vi "CRYExport TextFormat.vi"(8 "sAction":string, 11 "Type (data)":enum16{"data", "results"}(ring)) -> (0 "Canceled":bool, 3 "Export format":T1)   [LabVIEW 2013]
uses:
  CRYMainGlobal.vi
panel:
  out "Notation Frame":bool caption="符号"
  out "Layout Frame":bool caption="布局"
  out "Header":bool caption="页眉"
  out "Axes Saved":bool caption="保存的轴"
  in  "save z":bool
  in  "save y":bool
  in  "save x":bool
  in  "Comment":string caption="评论"
  in  "cancel":bool
  in  "save as":bool
  in  "Decimal places":i32=2 caption="小数位"
  in  "Custom Header":string caption="自定义页眉"
  in  "Character":string caption="字符"
  in  "Delimiter":i32(ring) caption="分隔符" items=["tab", "comma", "space", "other"]
  in  "notation":u16(slide) caption="Notation"
  in  "Layout":u16(slide)
  in  "Header format":u16(slide) caption="Header"
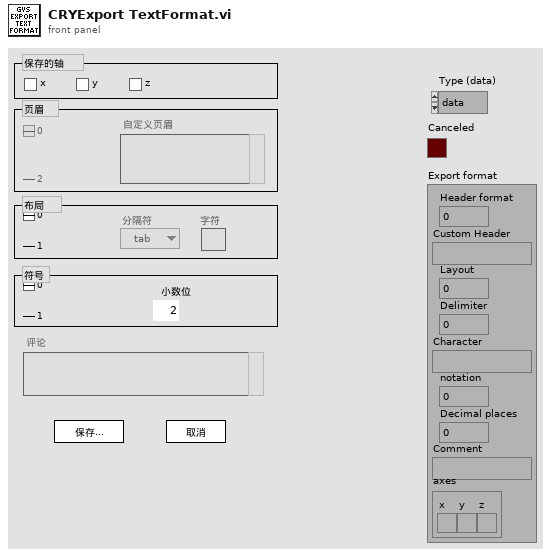
[diagram p1: front panel]
types:
  T1 = cluster{"Header format":u16, "Custom Header":string, "Layout":u16, "Delimiter":i32, "Character":string, "notation":u16, "Decimal places":i32, "Comment":string, "axes":cluster{"x":bool, "y":bool, "z":bool}}
  T2 = enum16{"open", "open or create", "create or replace", "create"}
  T3 = cluster{"Header format":u16, "Custom Header":string, "Layout":u16, "Delimiter":i32, "Character":string, "notation":u16, "Decimal places":i32, "Comment":string}
  T4 = enum8{"Enabled", "Disabled", "Disabled and Grayed Out"}
  T5 = cluster{"Header format":u16, "Custom Header":string, "Layout":u16, "Delimiter":i32, "Character":string, "notation":u16, "Decimal places":i32, "Comment":string, "axes":cluster{"x":bool, "y":bool, "z":bool}}[]
  T6 = cluster{"save x":bool, "save y":bool, "save z":bool}
  T7 = cluster{"Header format":u16, "Custom Header":string, "Layout":u16, "Delimiter":i32, "Character":string, "notation":u16, "Decimal places":i32, "Comment":string, cluster{"save x":bool, "save y":bool, "save z":bool}}
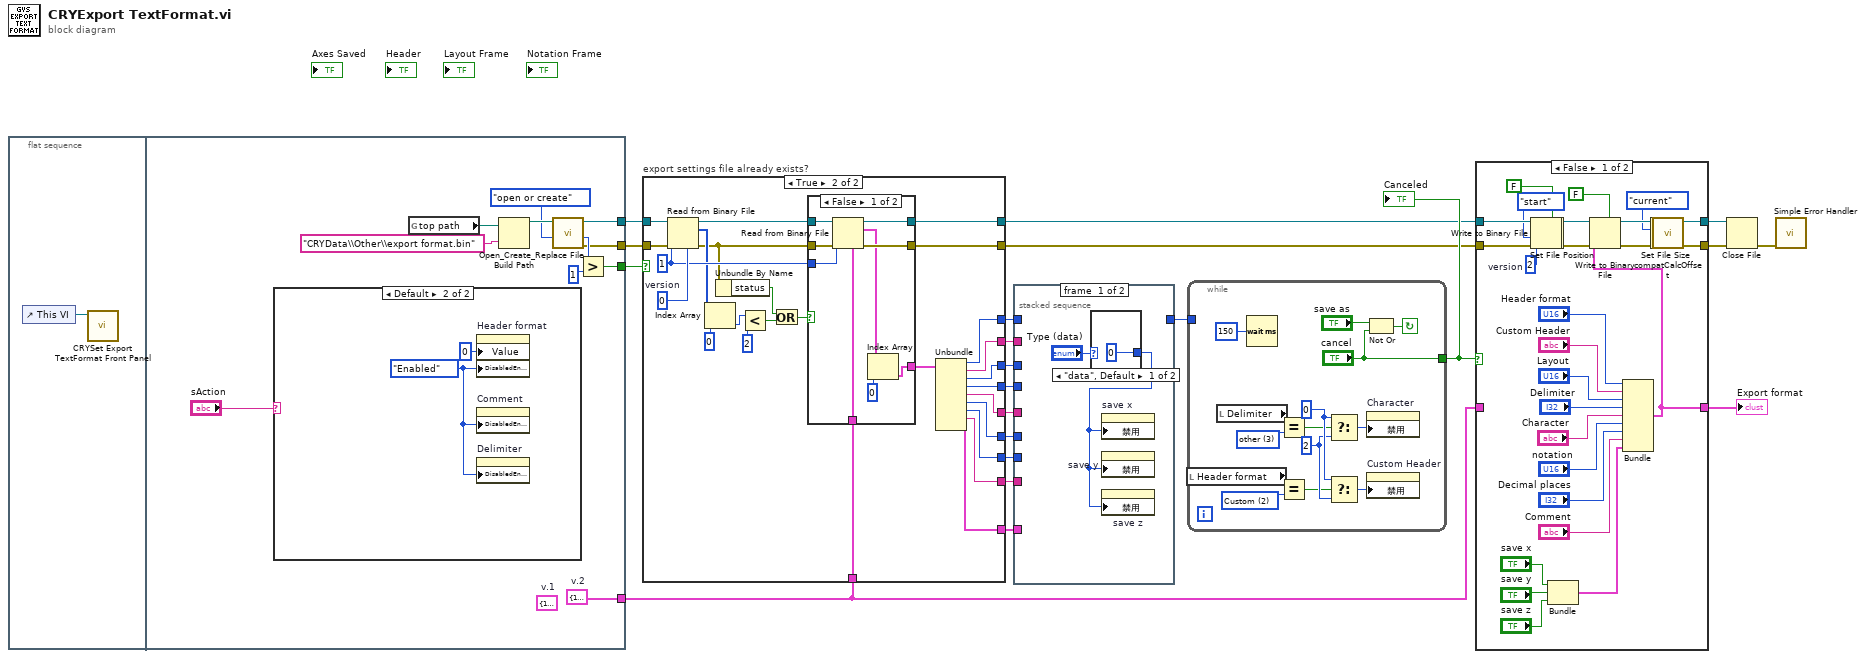
[diagram p0: block diagram]
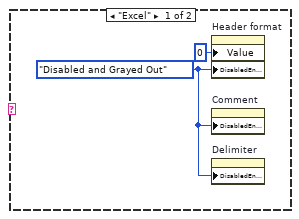
[diagram p2: hidden frame]
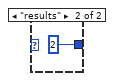
[diagram p4: hidden frame]
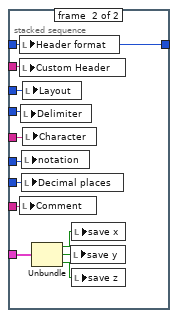
[diagram p5: hidden frame]
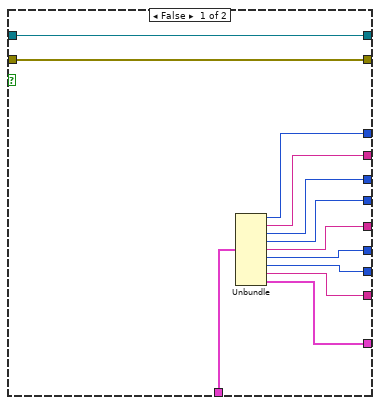
[diagram p6: hidden frame]
diagram:
  n1 = flat-sequence {
    tunnel: [w29] -> w21
    tunnel: [w28] -> w20
    tunnel: [w27] -> w19
    tunnel: [w26] -> w2
    frame #0 {
      n2 = control-ref of="This VI"() -> (w22:refnum<vi>)
      n3 = call "CRYSet Export TextFormat Front Panel.vi"("Vi Ref"=w22) -> ()  [unwired: 11 in]
    }
    frame #1 {
      w26 = T1 {"Header format"=1, "Custom Header"="", "Layout"=1, "Delimiter"=0, "Character"="", "notation"=0, "Decimal places"=4, "Comment"="", "axes"={"x"=TRUE, "y"=TRUE, "z"=FALSE}}  # v.2
      (unwired) T3 {"Header format"=1, "Custom Header"="", "Layout"=1, "Delimiter"=0, "Character"="", "notation"=0, "Decimal places"=4, "Comment"=""}  # v.1
      n4 = case shown="Default" "sAction" {
        frame "Excel" {
          w34 = T4."Disabled and Grayed Out" ("Disabled")
          n5 = property on="Header format" class="Slide (strict)"("Value"=u16 0 ("Header format"), "DisabledEnum"=w34) -> ()  [unwired: 2 in, 2 out]
          n6 = property on="Comment" class="Str"("DisabledEnum"=w34) -> ()  [unwired: 2 in, 2 out]
          n7 = property on="Delimiter" class="Ring (strict)"("DisabledEnum"=w34) -> ()  [unwired: 2 in, 2 out]
        }
        frame Default {
          w36 = T4."Enabled" ("Disabled")
          n8 = property on="Header format" class="Slide (strict)"("Value"=u16 0 ("Header format"), "DisabledEnum"=w36) -> ()  [unwired: 2 in, 2 out]
          n9 = property on="Comment" class="Str"("DisabledEnum"=w36) -> ()  [unwired: 2 in, 2 out]
          n10 = property on="Delimiter" class="Ring (strict)"("DisabledEnum"=w36) -> ()  [unwired: 2 in, 2 out]
        }
      }
      n11 = global read "CRYMainGlobal.vi" "top path"() -> (w24:path)
      n12 = Build Path(base path=w24, name or relative path="CRYData\\Other\\export format.bin") -> (appended path=w33:path)
      n13 = call <vilib>:"Open_Create_Replace File.vi"("function (open:0)"=T2."open or create", "file path"=w33) -> ("error out"=w28:errorcluster, "file size (bytes)"=w31:i32, "refnum"=w27:refnum<file>)  [unwired: 4 in, 3 out]
      n14 = Greater?(x=w31, y=1) -> (0:w29:bool)
    }
  }
  n15 = case "export settings file already exists?" shown="True" w21 {
    tunnel: w20 -> [w48 w74]
    tunnel: w19 -> [w49 w73]
    tunnel: [w48 w71] -> w17
    tunnel: [w49 w70] -> w16
    tunnel: [w43 w67] -> w12
    tunnel: [w46 w66] -> w11
    tunnel: [w40 w65] -> w10
    tunnel: [w41 w64] -> w9
    tunnel: [w42 w63] -> w8
    tunnel: [w45 w62] -> w7
    tunnel: [w44 w61] -> w6
    tunnel: w2 -> [w47 w60]
    tunnel: [w39 w59] -> w4
    tunnel: [w38 w58] -> w1
    frame False {
      n16 = Unbundle(w47) -> ("Header format"=w46:u16, "Custom Header"=w45:string, "Layout"=w44:u16, "Delimiter"=w43:i32, "Character"=w42:string, "notation"=w41:u16, "Decimal places"=w40:i32, "Comment"=w39:string, "axes"=w38:cluster{"x":bool, "y":bool, "z":bool})
    }
    frame True {
      w75 = u16 0  # version
      w69 = 1 ("count")
      n17 = Read from Binary File(5:w75, 8:w74, 10:w69, 11:w73) -> (0:w55:errorcluster, 2:w56:u16[], 3:w72:refnum<file>)  [unwired: 3 out]
      n18 = Index Array(array=w56, index=0 ("Index")) -> (element=w54:u16)
      n19 = Unbundle By Name(w55) -> ("status"=w51:bool)
      n20 = Less?(x=w54, y=u16 2 ("version")) -> (x < y?=w52:bool)
      n21 = Or(x=w51, y=w52) -> (x .or. y?=w50:bool)
      n22 = case shown="False" w50 {
        tunnel: w72 -> [w84 w87]
        tunnel: [w83 w86] -> w71
        tunnel: [w82 w87] -> w70
        tunnel: w69 -> [w81 _]
        tunnel: [w78 w85] -> w68
        tunnel: w60 -> [w77 w85]
        tunnel: w55 -> [w76 w86]
        frame False {
          n23 = Read from Binary File(5:w77, 8:w76, 10:w81, 11:w84) -> (0:w83:errorcluster, 2:w79:T5, 3:w82:refnum<file>)  [unwired: 3 out]
          n24 = Index Array(array=w79, index=0 ("Index")) -> (element=w78:T1)
        }
        frame True {
        }
      }
      n25 = Unbundle(w68) -> ("Header format"=w66:u16, "Custom Header"=w62:string, "Layout"=w61:u16, "Delimiter"=w67:i32, "Character"=w63:string, "notation"=w64:u16, "Decimal places"=w65:i32, "Comment"=w59:string, "axes"=w58:cluster{"x":bool, "y":bool, "z":bool})
    }
  }
  n26 = stacked-sequence {
    tunnel: [_ w102] -> w13
    tunnel: w12 -> [_ w103]
    tunnel: w11 -> [_ w102]
    tunnel: w10 -> [_ w101]
    tunnel: w9 -> [_ w100]
    tunnel: w8 -> [_ w99]
    tunnel: w7 -> [_ w98]
    tunnel: w6 -> [_ w97]
    tunnel: w4 -> [_ w96]
    tunnel: w1 -> [_ w95]
    frame #0 {
      n27 = case shown="\"data\", Default" "Type (data)" {
        tunnel: [u8 0 ("Write Attribute") u8 2 ("Write Attribute")] -> w88
        frame "data", Default {
        }
        frame "results" {
        }
      }
      n28 = property on="save x" class="Bool (strict)"("禁用"=w88) -> ()  [unwired: 2 in, 2 out]
      n29 = property on="save y" class="Bool (strict)"("禁用"=w88) -> ()  [unwired: 2 in, 2 out]
      n30 = property on="save z" class="Bool (strict)"("禁用"=w88) -> ()  [unwired: 2 in, 2 out]
    }
    frame #1 {
      n31 = local write "Header format"(w102) -> ()
      n32 = local write "Custom Header"(w98) -> ()
      n33 = local write "Comment"(w96) -> ()
      n34 = local write "Delimiter"(w103) -> ()
      n35 = local write "notation"(w100) -> ()
      n36 = local write "Decimal places"(w101) -> ()
      n37 = local write "Layout"(w97) -> ()
      n38 = local write "Character"(w99) -> ()
      n39 = Unbundle(w95) -> ("x"=w93:bool, "y"=w94:bool, "z"=w92:bool)
      n40 = local write "save y"(w94) -> ()
      n41 = local write "save x"(w93) -> ()
      n42 = local write "save z"(w92) -> ()
    }
  }
  n43 = while {
    tunnel: w13 -> [_]
    tunnel: ["cancel"] -> w18
    stop <- w116 continue-if-true
    w108 = u8 2 ("Write Attribute")
    w109 = u8 0 ("Write Attribute")
    w110 = u16 2 items=["None", "Standard", "Custom"] ("Header format")
    w112 = 3 items=["tab", "comma", "space", "other"] ("Delimiter")
    n44 = local read "Header format"() -> (w111:u16)
    n45 = local read "Delimiter"() -> (w113:i32)
    n46 = Wait (ms)(milliseconds to wait=u32 150) -> ()  [unwired: 1 out]
    n47 = Equal?(x=w113, y=w112) -> (x = y?=w106:bool)
    n48 = Equal?(x=w111, y=w110) -> (x = y?=w107:bool)
    n49 = Select(t=w109, s=w106, f=w108) -> (s? t:f=w105:u8)
    n50 = Select(t=w109, s=w107, f=w108) -> (s? t:f=w104:u8)
    n51 = Not Or(1:"cancel", 2:"save as") -> (0:w116:bool)
    n52 = property on="Character" class="Str"("禁用"=w105) -> ()  [unwired: 2 in, 2 out]
    n53 = property on="Custom Header" class="Str"("禁用"=w104) -> ()  [unwired: 2 in, 2 out]
  }
  "Canceled" <- w18
  n54 = case shown="False" w18 {
    tunnel: w17 -> [w141 w151]
    tunnel: w16 -> [w140 w150]
    tunnel: [w133 w151] -> w15
    tunnel: [w132 w150] -> w14
    tunnel: [w130 w149] -> w3
    tunnel: w2 -> [_ w149]
    frame False {
      w138 = u16 2  # version
      n55 = Set File Position(refnum=w140, from (0:start)=enum16{"start", "end", "current"}."start" ("pos mode (0:2)"), error in=w141) -> (refnum out=w120:refnum<file>, error out=w119:errorcluster)  [unwired: 1 out]
      n56 = Write to Binary File(file (use dialog)=w120, data=w138, error in=w119, 5:FALSE ("预置数组或字符串大小？(T)")) -> (refnum out=w136:refnum<file>, error out=w137:errorcluster)  [unwired: 3 out]
      n57 = Bundle("save x"="save x", "save y"="save y", "save z"="save z") -> (w125:T6)  [unwired: 1 out]
      n58 = Bundle("Header format"="Header format", "Custom Header"="Custom Header", "Layout"="Layout", "Delimiter"="Delimiter", "Character"="Character", "notation"="notation", "Decimal places"="Decimal places", "Comment"="Comment", w125) -> (w130:T7)  [unwired: 1 out]
      n59 = Write to Binary File(file (use dialog)=w136, data=w130, error in=w137, 5:FALSE ("预置数组或字符串大小？(T)")) -> (refnum out=w134:refnum<file>, error out=w135:errorcluster)  [unwired: 3 out]
      n60 = call <vilib>:"compatCalcOffset.vi"("error in"=w135, "pos mode (0:1)"=enum16{"start", "end", "current"}."current", "refnum"=w134) -> ("error out"=w124:errorcluster, "offset"=w123:i32, "dup refnum"=w122:refnum<file>)  [unwired: 1 in, 5 out]
      n61 = Set File Size(4:w124, 6:w123, 7:w122) -> (0:w133:errorcluster, 3:w132:refnum<file>)
    }
    frame True {
    }
  }
  "Export format" <- w3
  n62 = Close File(refnum=w14, error in=w15) -> (error out=w5:errorcluster)  [unwired: 1 out]
  n63 = call <vilib>:"Simple Error Handler.vi"("error in (no error)"=w5) -> ()  [unwired: 1 in, 8 out]
